vi "NivelMedidodB.vi"(8 "error in (no error)":errorcluster, 10 "voltaje_medido":dbl, 11 "Sensibilidad":dbl(knob)=0.1 scale=0.01..1.0 scale format="%#_6p") -> (0 "error out":errorcluster, 3 "Nivel Medido [dB]":dbl)   [LabVIEW 2019, in "Prueba09.lvclass"]
uses:
  Prueba09.lvclass
panel:
  out "voltaje mV":dbl
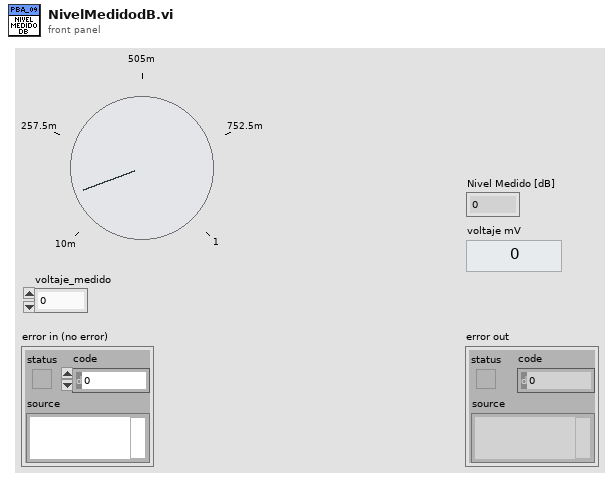
[diagram p1: front panel]
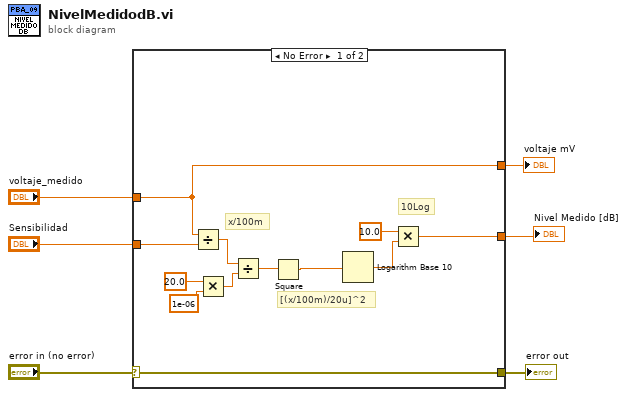
[diagram p0: block diagram]
diagram:
  n1 = case shown="No Error" "error in (no error)" {
    selector: "error in (no error)" -> [w8 w19]
    tunnel: [w8 w19] -> w5
    tunnel: [w10 _] -> w4
    tunnel: "Sensibilidad" -> [w9 _]
    tunnel: [w7 _] -> w2
    tunnel: "voltaje_medido" -> [w7 _]
    frame No Error {
      # "10Log"
      # "[(x/100m)/20u]^2"
      # "x/100m"
      n2 = Divide(x=w7, y=w9) -> (x/y=w18:dbl)
      n3 = Multiply(x=20.0, y=1e-06) -> (x*y=w15:dbl)
      n4 = Divide(x=w18, y=w15) -> (x/y=w14:dbl)
      n5 = Square(x=w14) -> (x^2=w11:dbl)
      n6 = Logarithm Base 10(1:w11) -> (0:w12:dbl)
      n7 = Multiply(x=10.0, y=w12) -> (x*y=w10:dbl)
    }
    frame Error {
    }
  }
  "error out" <- w5
  "Nivel Medido [dB]" <- w4
  "voltaje mV" <- w2
